vi "FSK - TESTBENCH2.vi"() -> ()   [LabVIEW 2013]
uses:
  Object/FSK_OBJ - PROP.ctl
  <vilib>/sound2/lvsound2.llb/Sampling Mode.ctl
  <vilib>/sound2/lvsound2.llb/Sound Data Format.ctl
  <vilib>/sound2/lvsound2.llb/Sound Output Write (DBL Single).vi
  <vilib>/Analysis/NI_AALPro.lvlib
  <vilib>/Analysis/NI_AALBase.lvlib
panel:
  in  "String":string="KD0QJP >> test"
  out "Array":u8[](array[numeric])
  out "x+y":dbl[](array[numeric])
  in  "PROPERTIES":T1={"rate (bit/s)"=128.0, "bp (Bit Period)"=1e-06, "f1%"=80.0, "f2%"=20.0, "f1 (1 Freq)"=0.0, "f2 (0 Freq)"=0.0, "t (Time arry)"=[], "y1 (f1 cos arry)"=[], "y2 (f2 cos arry)"=[], "data length (B)"=0, "data size"=0, "sample size"=0.0} {"f2%" format="%#_6f"; "f1%" format="%#_6f"; "sample size" format="%#_13g"; "y2 (f2 cos arry)" format="%#_6f"; "y1 (f1 cos arry)" format="%#_6f"; "t (Time arry)" format="%#_6f"; "f2 (0 Freq)" format="%#_6f"; "f1 (1 Freq)" format="%#_6f"; "bp (Bit Period)" format="%#_13f"; "rate (bit/s)" format="%#_13g"}
  in  "rate (bit/s)":dbl=128.0 format="%#_13g"
  out "x-y":u32=9198
  out "demodulated 2":dbl[](graph)
  in  "noise":dbl format="%#_13g"
  out "samples":dbl=344.53125 format="%#_13g"
  in  "data length (B)":i32=100
  out "demodulated":i16[][](graph)
  out "y1":dbl[](array[numeric])=[0.9893761484577952, 0.9577303262743624, 0.9057349344833171, 0.8344947557311932, 0.7455234801837959, 0.6407115430869976, 0.5222859573599328, 0.3927629946857276, 0.2548947205178964, 0.11161051901071738, -0.03404514966549826, -0.17897743711015687, -0.32010686511229053, -0.454434757489237, -0.5791069550678165, -0.6914744600109982, -0.789149720937414, -0.870057362904207, -0.9324782843576068, -0.9750861840923166, -0.9969757421057228, -0.9976818555685076, -0.9771895211914697, -0.9359341540109593, -0.8747923358194655, -0.7950631898159626, -0.6984407772219063, -0.5869781023713945, -0.46304349108464504, -0.32927026918416136, -0.18850081036952815, -0.04372614230499255, 0.10197760584826618, 0.24551456411120198, 0.38383490181300384, 0.5139996294876503, 0.6332430456494466, 0.7390315015970159, 0.8291172356286265, 0.901586132815433, 0.9548983955471564, 0.9879212606945145, 0.9999530682238599, 0.99073816986124, 0.9604723610310173, 0.9097987206528254, 0.8397939471916264, 0.7519454812884151, 0.6481199010631241, 0.5305232616169475, 0.40165422142856066, 0.26425095160066, 0.12123295601337575, -0.024360961427325113, -0.16943726439276915, -0.31091341467296013, -0.44578336903321847, -0.5711814507282928, -0.68444323855097, -0.7831621796627842, -0.8652407233141844, -0.928934888980065, -0.9728913219401479, -0.9961760489582477, -0.9982943230682821, -0.9792011358109098, -0.9393021735599112, -0.8794451976185704, -0.8009020312392202, -0.7053415363003983, -0.5947941538251642, -0.4716087617731102, -0.33840276677889497, -0.19800649027321907, -0.0534030306534317, 0.09233512070548741, 0.23611136283539147, 0.37487078083291553, 0.505665055784281, 0.6257151097701805, 0.7324701548882544, 0.8236618916370709, 0.8973527050704397, 0.9519768346644794, 0.9863736431323324, 0.9998122773006225, 0.992007197060682, 0.9631242424399986, 0.9137771098825537, 0.8450143126089946, 0.7582969021190435, 0.6554674242030396, 0.538710769076067, 0.4105077474793923, 0.27358237915042416, 0.13084401366014314, -0.014674486582761001, -0.15988118769183848, -0.30169078079605705, -0.4370901377666174, -0.5632023332687892, -0.6773477728172205, -0.7771011280039442, -0.8603428691562804, -0.9253043004739954, -0.9706051407525118, -0.9952828511881177, -0.9988130871166739, -0.9811208391333528, -0.9425820268702003, -0.884015511567408, -0.8066656971528188, -0.7121760895167505, -0.6025543757868123, -0.48012976558794696, -0.34750350068787894, -0.2074935845844053, -0.06307490640375905, 0.0826839686602312, 0.22668599930828476, 0.36587147314964674, 0.49728301856246626, 0.6181284420479548, 0.7258400559287772, 0.8181292358144563, 0.8930350486128749, 0.9489659178543944, 0.9847334410361209, 0.9995776404454229, 0.993183110940726, 0.9656857215863112, 0.917669728746776, 0.8501553619812785, 0.764577146508786, 0.6627534228421479, 0.5468477112287864, 0.41932274181484397, 0.2828881272862825, 0.14044278982303418, -0.004986634338720148, -0.1503101039746513, -0.2924398291507459, -0.4283558796669867, -0.5551703516376055, -0.6701887288153613, -0.7709671348727278, -0.8553642601604833, -0.9215868596193315, -0.9682278551184964, -0.9942962326340482, -0.9992380990206453, -0.9829484509686218, -0.9457734060831376, -0.8885028486800673, -0.8123536465585929, -0.7189437953555021, -0.6102580398543219, -0.48860570271744064, -0.3565716166838698, -0.2169612028106756, -0.07274086171932041, 0.07302505560394744, 0.21723935822802365, 0.35683782347021975, 0.4888543045900402, 0.6104837545943896, 0.719141827043265, 0.812519787475543, 0.8886335687133354, 0.9458659277322674, 0.9830008083610837, 0.99924917968211, 0.9942658011259113, 0.9681565580404066, 0.921476211870435, 0.8552166127512957, 0.7707856249715608, 0.6699772130907016, 0.5549333243127685, 0.42809837702819653, 0.29216732253760874, 0.15002838352677486, 0.004701685968533666, -0.14072491161716658, -0.28316142806424205, -0.4195814145628546, -0.547086259745096, -0.6629667785187164, -0.7647607760275437, -0.8503053636367329, -0.91778291534829, -0.9657596881785818, -0.9932162859035644, -0.9995693188870678, -0.9846837997705735, -0.9488760116445256, -0.8929067877591376, -0.8179653455653881, -0.7256440185757311, -0.617904422934397, -0.49703577758001233, -0.365606263601276, -0.22640845628773937, -0.0823999893192048, 0.06335928815654623, 0.20777232628990394, 0.34777067972510023, 0.48037970501603106, 0.6027817649670083, 0.71237609695127, 0.8068340731430783, 0.88414867851036, 0.9426771552741793, 0.9811759077382782, 0.9988269258411779, 0.9952551659910911, 0.9705365198808007, 0.9251962019635079, 0.8601975898520701, 0.7769217547575329, 0.6771381168980871, 0.5629668493836544, 0.4368338294071522, 0.3014190939261879, 0.15959989503350175, 0.014389564958840763, -0.13112651031957948, -0.27385644844022766, -0.41076756605667397, -0.5389508163928424, -0.6556825998051955, -0.7584826340192738, -0.8451666544310259, -0.9138928247125881, -0.9632008716036847, -0.9920431123643015, -0.999806715626468, -0.9863267226532054, -0.9518895523327884, -0.8972269154352526, -0.8235002674392077, -0.7322761302706873, -0.6254928073103707, -0.5054191988988894, -0.37460659341604435, -0.23583445826283292, -0.09205138256338727, 0.05368757358128155, 0.1982857921031729, 0.33867089298859904, 0.4718600152964715, 0.5950231961019138, 0.7055435007082523, 0.8010726264984068, 0.879580798971675, 0.939399899789645, 0.9792589104593589, 0.9983109185568722, 0.9961511126709647, 0.9728253837158201, 0.9288293498545073, 0.8650978257513989, 0.7829849599077564, 0.6842354621164354, 0.5709475323862405, 0.4455282790111326, 0.3106425730478823, 0.1691564259271335, 0.02407609329346504, -0.12151580102193553, -0.26452576367715097, -0.40191516144758455, -0.5307647852024573, -0.6483368763936876, -0.7521332981366267, -0.839948614880866, -0.9099169528499557, -0.9605516455734184, -0.990776822134496, -0.9999502669559449, -0.9878770654059384, -0.9548137452862886, -0.9014628262058824, -0.8289578926526208, -0.738839507926803, -0.633022480709521, -0.5137551797763668, -0.3835717613252466, -0.2452383239779305, -0.1016941355378064, 0.04401081969965071, 0.18878064610762815, 0.3295393173990277, 0.4632960351196873, 0.5872087762459463, 0.6986446796459717, 0.7952359883313769, 0.87493035885468, 0.9360344688935001, 0.9772499964605014, 0.9977012062634695, 0.9969535570687938, 0.9750229347045744, 0.9323753145232648, 0.8699168604957301, 0.7889746713082603, 0.6912685825637127, 0.5788746242252764, 0.45418090974819686, 0.31983689415418065, 0.17869707919773656, 0.033760361760447735, -0.11189368581954229, -0.2551702495862256, -0.393025031653726, -0.5225289345439073, -0.6409302977798866, -0.7457133643508318, -0.8346517347699798, -0.9058556729498477, -0.9578122587535489, -0.989417534072646, -0.9999999594012605, -0.9893346825080953, -0.9576483160298892, -0.905614122473395, -0.8343377089335418, -0.7453335354821389, -0.6404927363699581, -0.5220429377676673, -0.39250092582637613, -0.25461917075277707, -0.11132734313941778, 0.034329934806144054, 0.1792577804900378, 0.32037681007850216, 0.4546885683312952, 0.5793392388883094, 0.691680281312277, 0.7893247064895802, 0.8701977946662005, 0.9325811784770495, 0.9751493543055092, 0.9969978461907315, 0.9976624238642972]
  out "y2":dbl[](array[numeric])=[0.999334903985156, 0.997340500646042, 0.9940194429220834, 0.9893761484577952, 0.983416793726465, 0.9761493058142584, 0.9675833518756722, 0.9577303262743624, 0.9466033354264518, 0.9342171803664809, 0.920588337059189, 0.9057349344833171, 0.8896767305165856, 0.8724350856539221, 0.8540329345939015, 0.8344947557311932, 0.8138465385955947, 0.7921157492809673, 0.769331293910056, 0.7455234801837959, 0.7207239770662501, 0.6949657726588057, 0.6682831303196646, 0.6407115430869973, 0.6122876864663866, 0.5830493696453622, 0.5530354851999211, 0.5222859573599322, 0.49084168890224517, 0.458744506742142, 0.4260371062955071, 0.3927629946857266, 0.3589664328708588, 0.3246923767680605, 0.2899864174535852, 0.25489472051789513, 0.21946396465656262, 0.1837412795786402, 0.1477741833150976, 0.11161051901071582, 0.07529839128351644, 0.0388861022363834, 0.002422087205989877, -0.034045149665500256, -0.07046709995025559, -0.10679531546030208, -0.14298147269291528, -0.1789774371101593, -0.2147353271670654, -0.2502075780032812, -0.2853470047134697, -0.320106865112293, -0.3544409219104956, -0.3883035042193773, -0.4216495683018469, -0.4544347574892398, -0.4866154611842069, -0.5181488728711843, -0.5489930470572765, -0.5791069550678191, -0.6084505396223935, -0.6369847681187029, -0.6646716845534281, -0.6914744600110011, -0.7173574416531345, -0.7422862001439438, -0.7662275754475737, -0.7891497209374164, -0.8110221457582377, -0.831815755384871, -0.8515028903235224, -0.8700573629042091, -0.8874544921153893, -0.9036711364344469, -0.9186857246103601, -0.9324782843576086, -0.9450304689231472, -0.9563255814911122, -0.966348597392791, -0.9750861840923176, -0.9825267189215059, -0.9886603045402291, -0.9934787821017842, -0.9969757421057232, -0.9991465329237209, -0.9999882669871332, -0.9994998246280177, -0.9976818555685074, -0.9945367780565556, -0.9900687756492015, -0.9842837916476358, -0.9771895211914694, -0.9687954010227195, -0.9591125969331309, -0.9481539889115284, -0.9359341540109589, -0.9224693469584113, -0.9077774785329082, -0.8918780917407305, -0.8747923358194658, -0.856542938105462, -0.8371541738021047, -0.8166518336891359, -0.7950631898159637, -0.7724169592246001, -0.7487432657504801, -0.7240735999519763, -0.6984407772219086, -0.6718788941367715, -0.6444232831017385, -0.6161104653517774, -0.5869781023713981, -0.5570649457976438, -0.5264107858729701, -0.4950563985165871, -0.4630434910846506, -0.4304146468914752, -0.39721326856554295, -0.3634835203156785, -0.3292702691841681, -0.2946190253649748, -0.25957588166644746, -0.22418745219902733, -0.18850081036953686, -0.15256342626450223, -0.11642310350582868, -0.08012791566280102, -0.043726142305002304, -0.00726620478122136, 0.029203398190246532, 0.06563415503420107, 0.1019776058482547, 0.13818540686380232, 0.17420939475251962, 0.21000165069284124, 0.24551456411118905, 0.2807008960131847, 0.3155138418205765, 0.3499070936303232, 0.38383490181299157, 0.41725213586855137, 0.4501143444586093, 0.4823778145352195, 0.5139996294876373, 0.5449377262296482, 0.5751509511515512, 0.6045991148623658, 0.6332430456494335, 0.6610446415843235, 0.6879669212057095, 0.7139740727118193, 0.7390315015970039, 0.7631058766690754, 0.7861651743861942, 0.8081787214543256, 0.8291172356286155, 0.8489528646643949, 0.8676592233660174, 0.8852114286842332, 0.9015861328154241, 0.9167615542586671, 0.9307175067893105, 0.943435426310532, 0.9548983955471497, 0.9650911665488493, 0.9740001809728829, 0.9816135881192718, 0.9879212606945109, 0.9929148082828151, 0.9965875885069823, 0.9989347158640314, 0.9999530682238595, 0.9996412909822744, 0.9979997988628776, 0.9950307753654032, 0.9907381698612435, 0.9851276923400267, 0.9782068058142344, 0.9699847163919613, 0.9604723610310247, 0.9496823929907088, 0.9376291650005016, 0.9243287101682082, 0.9097987206528368, 0.8940585241306331, 0.8771290580855559, 0.8590328419584059, 0.8397939471916422, 0.8194379652097441, 0.7979919733777007, 0.7754844989829147, 0.7519454812884356, 0.7274062317079862, 0.7018993921557741, 0.675458891626473, 0.6481199010631484, 0.6199187865731481, 0.5908930610541938, 0.5610813342950279, 0.5305232616169754, 0.49925949112475654, 0.4673316096366968, 0.43478208736627705, 0.40165422142859236, 0.367992078246872, 0.3338404349356802, 0.2992447197387486, 0.2642509516006951, 0.22890567895298405, 0.1932559177955794, 0.15734908915663393, 0.12123295601341277, 0.08495555975836794, 0.04856515629485395, 0.012110151847516893, -0.024360961427286932, -0.06079966994536465, -0.09715750322707249, -0.13338609837236418, -0.1694372643927289, -0.20526304631446715, -0.24081578896800843, -0.2760482003784414, -0.3109134146729196, -0.3453650544212785, -0.37935729232691345, -0.41284491218589114, -0.44578336903318033, -0.4781288483960157, -0.5098383245755508, -0.5408696178793061, -0.5711814507282579, -0.6007335025639439, -0.6294864634825542, -0.6574020865246436, -0.6844432385509376, -0.7105739496365373, -0.7357594609178254, -0.7599662708284343, -0.7831621796627555, -0.8053163324077363, -0.8263992597859696, -0.8463829174554968, -0.8652407233141605, -0.8829475928589102, -0.8994799725530068, -0.9148158711567487, -0.9289348889800466, -0.9418182450179241, -0.9534488019328641, -0.9638110888507574, -0.9728913219401361, -0.9806774227473178, -0.9871590342630662, -0.9923275346994032, -0.9961760489582432, -0.9986994577765927, -0.9998944045361543, -0.9997592997282723, -0.9982943230682852, -0.9955014232564702, -0.9913843153858962, -0.9859484760006382, -0.979201135810921, -0.9711512700748869, -0.9618095866597781, -0.9511885117984167, -0.9393021735599301, -0.9261663830567055, -0.911798613412574, -0.8962179765202013, -0.8794451976185975, -0.8615025877245741, -0.8424140139548039, -0.8222048677779745, -0.8009020312392553, -0.7785338412020207, -0.7551300516543767, -0.7307217941306443, -0.7053415363004412, -0.6790230387804421, -0.6518013102262827, -0.6237125607643202, -0.5947941538252127, -0.5650845564433834, -0.5346232880884718, -0.5034508680968593, -0.471608761773165, -0.4391393252334305, -0.40608574906334644, -0.37249200086648837, -0.33840276677895514, -0.3038633920282282, -0.2689198206153131, -0.23361853420038867, -0.1980064902732835, -0.1621310596909903, -0.12603996366533124, -0.0897812102845842, -0.053403030653499106, -0.016953814736677533, 0.019517953009379575, 0.05596375812990778, 0.09233512070541842, 0.12858365983930822, 0.16466115801373166, 0.20051962522816602, 0.23611136283532413, 0.27138902698952166, 0.306305691623073, 0.3408149108669792, 0.3748707808328513, 0.40842800067389506, 0.4414419328437426, 0.47386866247295134, 0.5056650557842197, 0.5367888174685921, 0.5671985469463406, 0.5968537934376921, 0.6257151097701237, 0.6537441048506837, 0.6809034947335145, 0.7071571522146655, 0.7324701548882036, 0.7568088315997251, 0.7801408072354551, 0.8024350457873651, 0.8236618916370276, 0.8437931090032768, 0.8628019195012241, 0.8806630377626514, 0.8973527050704053, 0.9128487209620563, 0.9271304727607728, 0.9401789629941419, 0.9519768346644555, 0.9625083943368513, 0.9717596330145924, 0.9797182447737252, 0.9863736431323198, 0.9917169751325254, 0.9957411331167036, 0.9984407641819776, 0.999812277300621, 0.9998538480968151]
  out "size(s)":i32=276000
  out "m":dbl[](graph)
  out "t2":dbl[](array[numeric])=[2.9024943310657594e-09, 5.804988662131519e-09, 8.707482993197278e-09, 1.1609977324263038e-08, 1.4512471655328797e-08, 1.7414965986394556e-08, 2.0317460317460316e-08, 2.3219954648526075e-08, 2.6122448979591834e-08, 2.9024943310657594e-08, 3.192743764172335e-08, 3.482993197278911e-08, 3.773242630385487e-08, 4.063492063492063e-08, 4.353741496598639e-08, 4.643990929705215e-08, 4.934240362811791e-08, 5.224489795918367e-08, 5.514739229024943e-08, 5.804988662131519e-08, 6.095238095238095e-08, 6.385487528344672e-08, 6.675736961451249e-08, 6.965986394557825e-08, 7.256235827664402e-08, 7.546485260770978e-08, 7.836734693877555e-08, 8.126984126984132e-08, 8.417233560090708e-08, 8.707482993197285e-08, 8.997732426303861e-08, 9.287981859410438e-08, 9.578231292517015e-08, 9.868480725623591e-08, 1.0158730158730168e-07, 1.0448979591836744e-07, 1.0739229024943321e-07, 1.1029478458049898e-07, 1.1319727891156474e-07, 1.1609977324263051e-07, 1.1900226757369627e-07, 1.2190476190476204e-07, 1.248072562358278e-07, 1.2770975056689357e-07, 1.3061224489795934e-07, 1.335147392290251e-07, 1.3641723356009087e-07, 1.3931972789115664e-07, 1.422222222222224e-07, 1.4512471655328817e-07, 1.4802721088435393e-07, 1.509297052154197e-07, 1.5383219954648547e-07, 1.5673469387755123e-07, 1.59637188208617e-07, 1.6253968253968276e-07, 1.6544217687074853e-07, 1.683446712018143e-07, 1.7124716553288006e-07, 1.7414965986394583e-07, 1.770521541950116e-07, 1.7995464852607736e-07, 1.8285714285714313e-07, 1.857596371882089e-07, 1.8866213151927466e-07, 1.9156462585034042e-07, 1.944671201814062e-07, 1.9736961451247196e-07, 2.0027210884353772e-07, 2.031746031746035e-07, 2.0607709750566925e-07, 2.0897959183673502e-07, 2.1188208616780079e-07, 2.1478458049886655e-07, 2.1768707482993232e-07, 2.2058956916099808e-07, 2.2349206349206385e-07, 2.2639455782312962e-07, 2.2929705215419538e-07, 2.3219954648526115e-07, 2.3510204081632691e-07, 2.3800453514739268e-07, 2.4090702947845845e-07, 2.438095238095242e-07, 2.467120181405899e-07, 2.4961451247165566e-07, 2.525170068027214e-07, 2.5541950113378714e-07, 2.583219954648529e-07, 2.612244897959186e-07, 2.6412698412698436e-07, 2.670294784580501e-07, 2.6993197278911584e-07, 2.728344671201816e-07, 2.757369614512473e-07, 2.7863945578231306e-07, 2.815419501133788e-07, 2.8444444444444454e-07, 2.873469387755103e-07, 2.90249433106576e-07, 2.9315192743764176e-07, 2.960544217687075e-07, 2.9895691609977324e-07, 3.01859410430839e-07, 3.047619047619047e-07, 3.0766439909297045e-07, 3.105668934240362e-07, 3.1346938775510193e-07, 3.1637188208616767e-07, 3.192743764172334e-07, 3.2217687074829915e-07, 3.250793650793649e-07, 3.2798185941043063e-07, 3.3088435374149637e-07, 3.337868480725621e-07, 3.3668934240362785e-07, 3.395918367346936e-07, 3.4249433106575933e-07, 3.4539682539682507e-07, 3.482993197278908e-07, 3.5120181405895655e-07, 3.541043083900223e-07, 3.5700680272108803e-07, 3.5990929705215377e-07, 3.628117913832195e-07, 3.6571428571428525e-07, 3.68616780045351e-07, 3.715192743764167e-07, 3.7442176870748246e-07, 3.773242630385482e-07, 3.8022675736961394e-07, 3.831292517006797e-07, 3.860317460317454e-07, 3.8893424036281116e-07, 3.918367346938769e-07, 3.9473922902494264e-07, 3.976417233560084e-07, 4.005442176870741e-07, 4.0344671201813986e-07, 4.063492063492056e-07, 4.0925170068027134e-07, 4.121541950113371e-07, 4.150566893424028e-07, 4.1795918367346856e-07, 4.208616780045343e-07, 4.2376417233560004e-07, 4.266666666666658e-07, 4.295691609977315e-07, 4.3247165532879725e-07, 4.35374149659863e-07, 4.3827664399092873e-07, 4.4117913832199447e-07, 4.440816326530602e-07, 4.4698412698412595e-07, 4.498866213151917e-07, 4.5278911564625743e-07, 4.5569160997732317e-07, 4.585941043083889e-07, 4.6149659863945465e-07, 4.643990929705204e-07, 4.6730158730158613e-07, 4.7020408163265187e-07, 4.731065759637176e-07, 4.7600907029478335e-07, 4.789115646258491e-07, 4.818140589569149e-07, 4.847165532879806e-07, 4.876190476190464e-07, 4.905215419501121e-07, 4.934240362811778e-07, 4.963265306122436e-07, 4.992290249433093e-07, 5.021315192743751e-07, 5.050340136054408e-07, 5.079365079365065e-07, 5.108390022675723e-07, 5.13741496598638e-07, 5.166439909297038e-07, 5.195464852607695e-07, 5.224489795918352e-07, 5.25351473922901e-07, 5.282539682539667e-07, 5.311564625850325e-07, 5.340589569160982e-07, 5.369614512471639e-07, 5.398639455782297e-07, 5.427664399092954e-07, 5.456689342403611e-07, 5.485714285714269e-07, 5.514739229024926e-07, 5.543764172335584e-07, 5.572789115646241e-07, 5.601814058956898e-07, 5.630839002267556e-07, 5.659863945578213e-07, 5.688888888888871e-07, 5.717913832199528e-07, 5.746938775510185e-07, 5.775963718820843e-07, 5.8049886621315e-07, 5.834013605442158e-07, 5.863038548752815e-07, 5.892063492063472e-07, 5.92108843537413e-07, 5.950113378684787e-07, 5.979138321995445e-07, 6.008163265306102e-07, 6.037188208616759e-07, 6.066213151927417e-07, 6.095238095238074e-07, 6.124263038548732e-07, 6.153287981859389e-07, 6.182312925170046e-07, 6.211337868480704e-07, 6.240362811791361e-07, 6.269387755102019e-07, 6.298412698412676e-07, 6.327437641723333e-07, 6.356462585033991e-07, 6.385487528344648e-07, 6.414512471655306e-07, 6.443537414965963e-07, 6.47256235827662e-07, 6.501587301587278e-07, 6.530612244897935e-07, 6.559637188208593e-07, 6.58866213151925e-07, 6.617687074829907e-07, 6.646712018140565e-07, 6.675736961451222e-07, 6.70476190476188e-07, 6.733786848072537e-07, 6.762811791383194e-07, 6.791836734693852e-07, 6.820861678004509e-07, 6.849886621315166e-07, 6.878911564625824e-07, 6.907936507936481e-07, 6.936961451247139e-07, 6.965986394557796e-07, 6.995011337868453e-07, 7.024036281179111e-07, 7.053061224489768e-07, 7.082086167800426e-07, 7.111111111111083e-07, 7.14013605442174e-07, 7.169160997732398e-07, 7.198185941043055e-07, 7.227210884353713e-07, 7.25623582766437e-07, 7.285260770975027e-07, 7.314285714285685e-07, 7.343310657596342e-07, 7.372335600907e-07, 7.401360544217657e-07, 7.430385487528314e-07, 7.459410430838972e-07, 7.488435374149629e-07, 7.517460317460287e-07, 7.546485260770944e-07, 7.575510204081601e-07, 7.604535147392259e-07, 7.633560090702916e-07, 7.662585034013574e-07, 7.691609977324231e-07, 7.720634920634888e-07, 7.749659863945546e-07, 7.778684807256203e-07, 7.80770975056686e-07, 7.836734693877518e-07, 7.865759637188175e-07, 7.894784580498833e-07, 7.92380952380949e-07, 7.952834467120147e-07, 7.981859410430805e-07, 8.010884353741462e-07, 8.03990929705212e-07, 8.068934240362777e-07, 8.097959183673434e-07, 8.126984126984092e-07, 8.156009070294749e-07, 8.185034013605407e-07, 8.214058956916064e-07, 8.243083900226721e-07, 8.272108843537379e-07, 8.301133786848036e-07, 8.330158730158694e-07, 8.359183673469351e-07, 8.388208616780008e-07, 8.417233560090666e-07, 8.446258503401323e-07, 8.475283446711981e-07, 8.504308390022638e-07, 8.533333333333295e-07, 8.562358276643953e-07, 8.59138321995461e-07, 8.620408163265268e-07, 8.649433106575925e-07, 8.678458049886582e-07, 8.70748299319724e-07, 8.736507936507897e-07, 8.765532879818555e-07, 8.794557823129212e-07, 8.823582766439869e-07, 8.852607709750527e-07, 8.881632653061184e-07, 8.910657596371842e-07, 8.939682539682499e-07, 8.968707482993156e-07, 8.997732426303814e-07, 9.026757369614471e-07, 9.055782312925129e-07, 9.084807256235786e-07, 9.113832199546443e-07, 9.142857142857101e-07, 9.171882086167758e-07, 9.200907029478415e-07, 9.229931972789073e-07, 9.25895691609973e-07, 9.287981859410388e-07, 9.317006802721045e-07, 9.346031746031702e-07, 9.37505668934236e-07, 9.404081632653017e-07, 9.433106575963675e-07, 9.462131519274332e-07, 9.491156462584989e-07, 9.520181405895647e-07, 9.549206349206304e-07, 9.578231292516962e-07, 9.60725623582762e-07, 9.636281179138276e-07, 9.665306122448934e-07, 9.694331065759591e-07, 9.723356009070249e-07, 9.752380952380906e-07, 9.781405895691563e-07, 9.81043083900222e-07, 9.839455782312878e-07, 9.868480725623536e-07, 9.897505668934193e-07, 9.92653061224485e-07, 9.955555555555508e-07, 9.984580498866165e-07, 1.0013605442176823e-06] format="%#_6f"
  out "ss":i32=345
  out "f2 (0 Freq)":dbl=2000000.0 format="%#_6f"
  out "f1 (1 Freq)":dbl=8000000.0 format="%#_6f"
  out "br (Bit Rate)":dbl=1000000.0 format="%#_6f"
  in  "bp (Bit Period)":dbl=1e-06 format="%#_13f"
  # "ss=700, data=100, time=25000 rate=32 bit/s\nss=700, data=50,   time=13000 rate=31 bit/s \nss=440, data=100, time=8000   rate=100 bit/s\nss=100, data=100, time=2000   rate=400 bit/s\nss=10000, data=100, time=183000, rate=4.3 bit/s\nss=1000, data=100, time=18500, rate=43 bit/s"
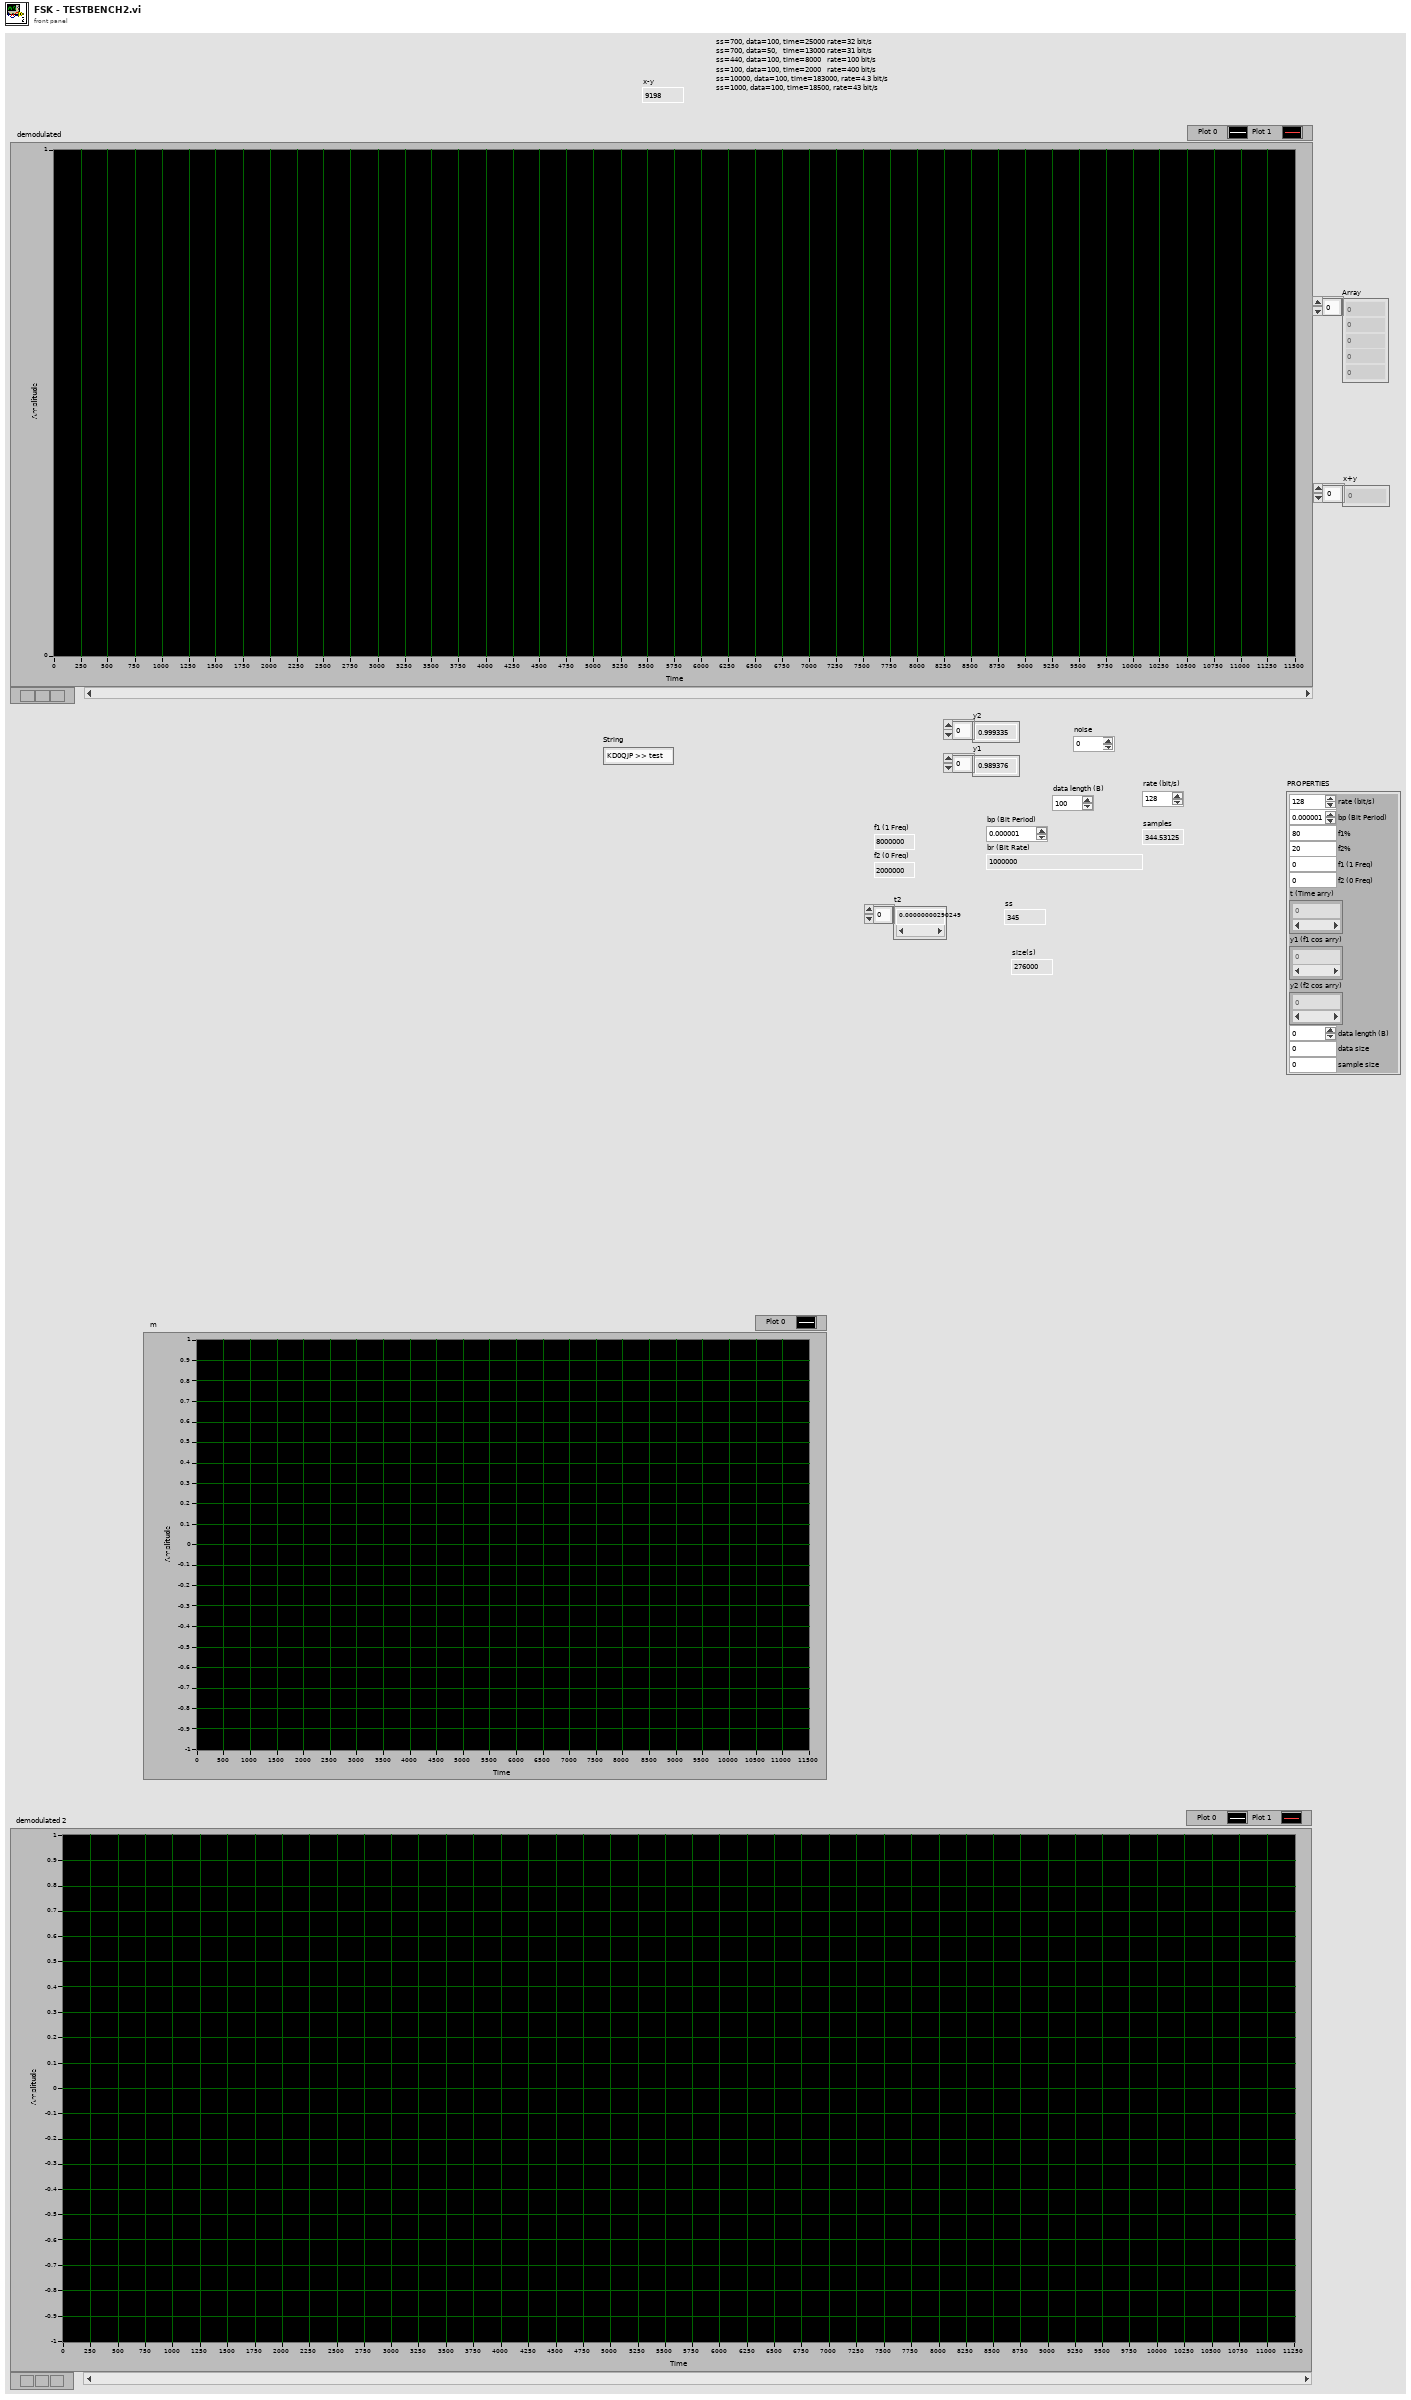
[diagram p1: front panel]
types:
  T1 = typedef "FSK_OBJ - PROP.ctl" = cluster{"rate (bit/s)":dbl, "bp (Bit Period)":dbl, "f1%":dbl, "f2%":dbl, "f1 (1 Freq)":dbl, "f2 (0 Freq)":dbl, "t (Time arry)":dbl[], "y1 (f1 cos arry)":dbl[], "y2 (f2 cos arry)":dbl[], "data length (B)":i32, "data size":i32, "sample size":dbl}
  T2 = typedef "Sound Data Format.ctl" = cluster{"sample rate (S/s)":dbl, "number of channels":i32, "bits per sample":i32}
  T3 = typedef "Sampling Mode.ctl" = i32
  T4 = typedef "Sound Output Task ID.ctl" = u32
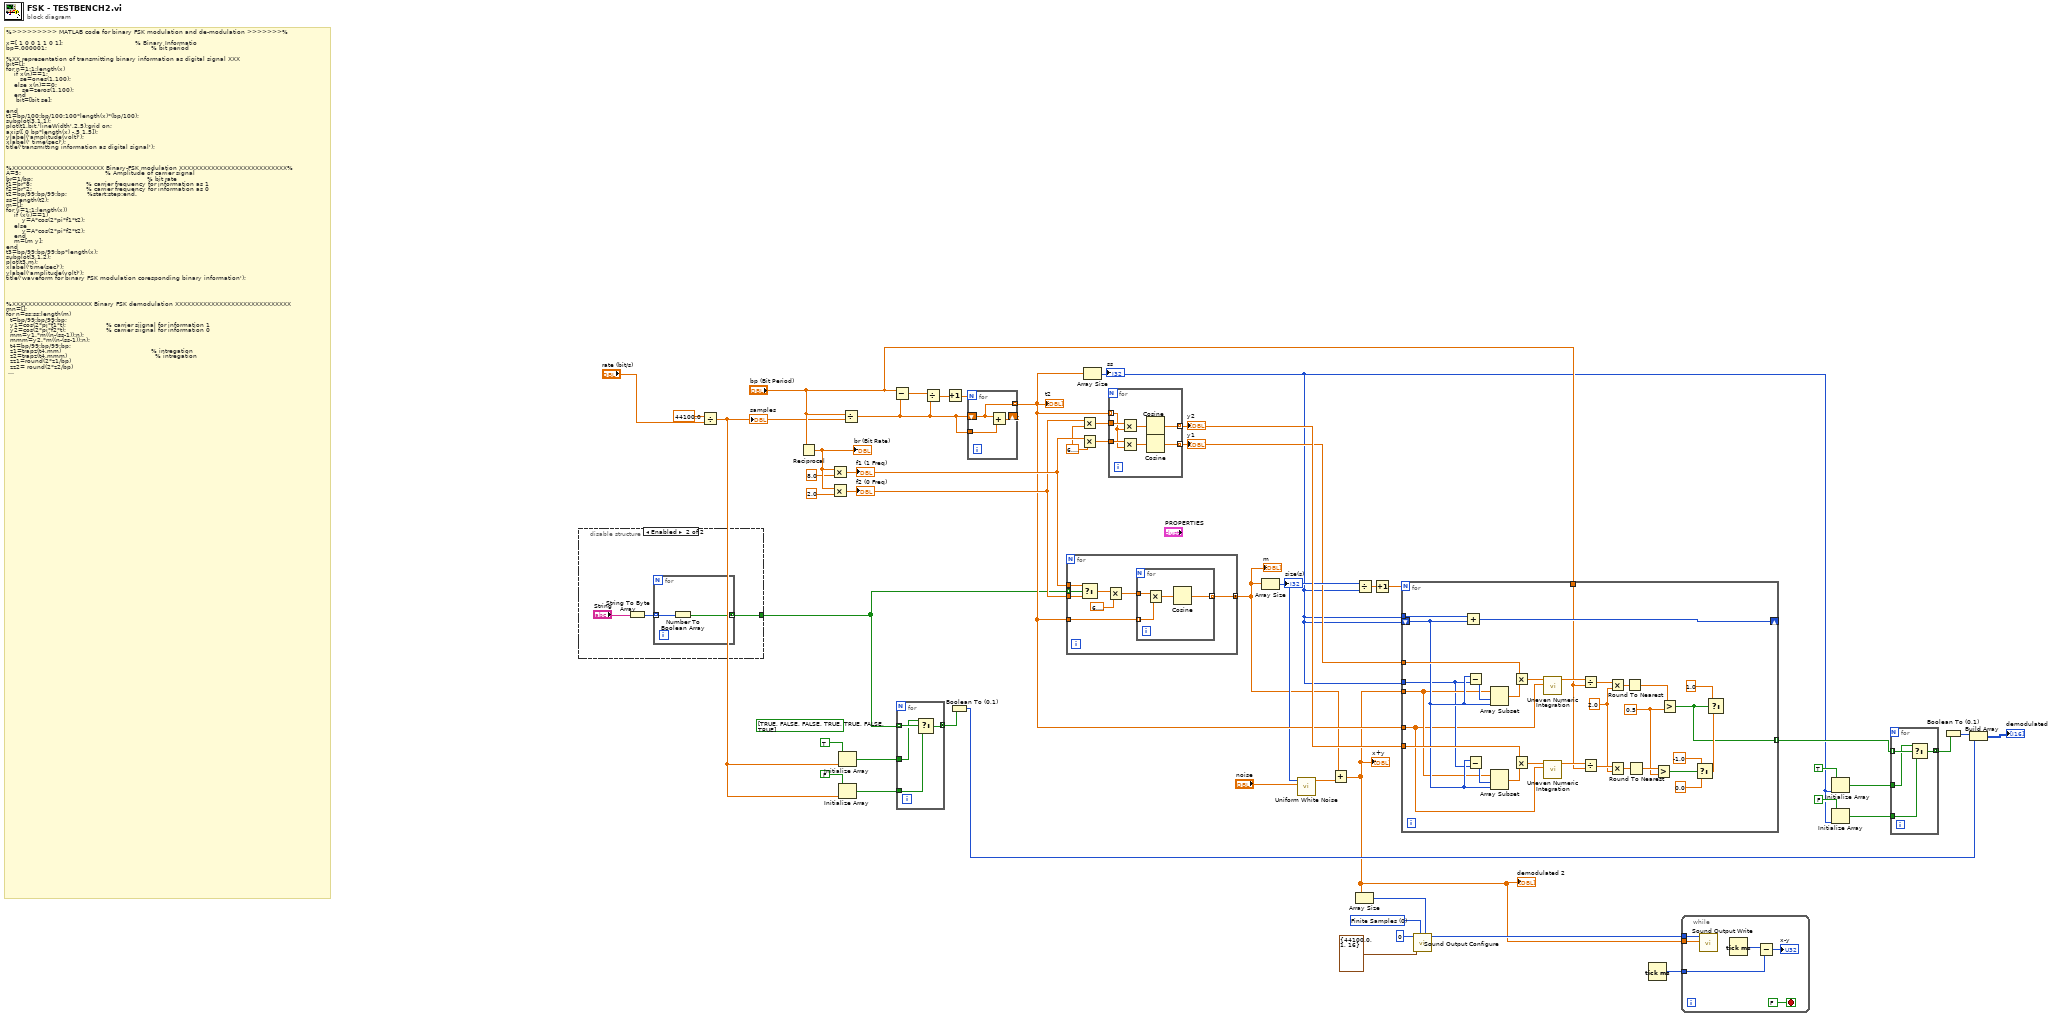
[diagram p0: block diagram]
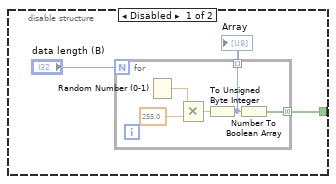
[diagram p2: hidden frame]
diagram:
  w23 = T3 0 items=["Finite Samples", "Continuous Samples"] ("sample mode")
  w34 = 6.283185307179586
  (unwired) bool[] [TRUE, FALSE, FALSE, TRUE, TRUE, FALSE, TRUE]
  # "%>>>>>>>>> MATLAB code for binary FSK modulation and de-modulation >>>>>>>%\n\nx=[ 1 0 0 1 1 0 1];                                    % Binary Informatio\nbp=.000001;                                                    % bit period\n\n%XX representation of transmitting binary information as digital signal XXX\nbit=[]; \nfor n=1:1:length(x)\n    if x(n)==1;\n       se=ones(1,100);\n    else x(n)==0;\n        se=zeros(1,100);\n    end\n     bit=[bit se];\n\nend\nt1=bp/100:bp/100:100*length(x)*(bp/100);\nsubplot(3,1,1);\nplot(t1,bit,'lineWidth',2.5);grid on;\naxis([ 0 bp*length(x) -.5 1.5]);\nylabel('amplitude(volt)');\nxlabel(' time(sec)');\ntitle('transmitting information as digital signal');\n\n\n\n%XXXXXXXXXXXXXXXXXXXXXXX Binary-FSK modulation XXXXXXXXXXXXXXXXXXXXXXXXXXX%\nA=5;                                          % Amplitude of carrier signal\nbr=1/bp;                                                         % bit rate\nf1=br*8;                           % carrier frequency for information as 1\nf2=br*2;                           % carrier frequency for information as 0\nt2=bp/99:bp/99:bp;          %start:step:end.       \nss=length(t2);\nm=[];\nfor (i=1:1:length(x))\n    if (x(i)==1)\n        y=A*cos(2*pi*f1*t2);\n    else\n        y=A*cos(2*pi*f2*t2);\n    end\n    m=[m y];\nend\nt3=bp/99:bp/99:bp*length(x);\nsubplot(3,1,2);\nplot(t3,m);\nxlabel('time(sec)');\nylabel('amplitude(volt)');\ntitle('waveform for binary FSK modulation coresponding binary information');\n\n\n\n\n%XXXXXXXXXXXXXXXXXXXX Binary FSK demodulation XXXXXXXXXXXXXXXXXXXXXXXXXXXXX\nmn=[];\nfor n=ss:ss:length(m)\n  t=bp/99:bp/99:bp;\n  y1=cos(2*pi*f1*t);                    % carrier siignal for information 1\n  y2=cos(2*pi*f2*t);                    % carrier siignal for information 0\n  mm=y1.*m((n-(ss-1)):n);\n  mmm=y2.*m((n-(ss-1)):n);\n  t4=bp/99:bp/99:bp;\n  z1=trapz(t4,mm)                                             % intregation \n  z2=trapz(t4,mmm)                                            % intregation \n  zz1=round(2*z1/bp)\n  zz2= round(2*z2/bp)\n  if(zz1>A/2)      % logic lavel= (0+A)/2 or (A+0)/2 or 2.5 ( in this case)\n    a=1;\n  else(zz2>A/2)\n    a=0;\n  end\n  mn=[mn a];\nend\ndisp(' Binary information at Reciver :');\ndisp(mn);\n\n\n%XXXXX Representation of binary information as digital signal which achived \n%after demodulation XXXXXXXXXXXXXXXXXXXXXXXXXXXXXXXXXXXXXXXXXXXXXXXXXXXXXXX\nbit=[];\nfor n=1:length(mn);\n    if mn(n)==1;\n       se=ones(1,100);\n    else mn(n)==0;\n        se=zeros(1,100);\n    end\n     bit=[bit se];\n\nend\nt4=bp/100:bp/100:100*length(mn)*(bp/100);\nsubplot(3,1,3)\nplot(t4,bit,'LineWidth',2.5);grid on;\naxis([ 0 bp*length(mn) -.5 1.5]);\nylabel('amplitude(volt)');\nxlabel(' time(sec)');\ntitle('recived information as digital signal after binary FSK demodulation');\n\n\n\n%>>>>>>>>>>>>>>>>>>>>>>>>>> end of program >>>>>>>>>>>>>>>>>>>>>>>>>>>>>>%"
  n1 = disable-structure shown="Enabled" {
    disable-tunnel: [w50 w57] -> w13
    frame Disabled {
      n2 = for {
        N: "data length (B)" -> [_]
        tunnel: [w53] -> w50 mode=concatenating
        tunnel: [w52] -> w49 mode=indexing
        n3 = Random Number (0-1)() -> (number: 0 to 1=w56:dbl)
        n4 = Multiply(x=w56, y=255.0) -> (x*y=w54:dbl)
        n5 = To Unsigned Byte Integer(number=w54) -> (unsigned 8bit integer=w52:u8)
        n6 = Number To Boolean Array(number=w52) -> (Boolean array=w53:bool[])
      }
      "Array" <- w49
    }
    frame Enabled {
      n7 = String To Byte Array(string="String") -> (unsigned byte array=w58:u8[])
      n8 = for {
        tunnel: w58 -> [w61] mode=indexing
        tunnel: [w60] -> w57 mode=concatenating
        n9 = Number To Boolean Array(number=w61) -> (Boolean array=w60:bool[])
      }
    }
  }
  n10 = Divide(x=44100.0, y="rate (bit/s)") -> (x/y=w6:dbl)
  "samples" <- w6
  n11 = Reciprocal(x="bp (Bit Period)") -> (1/x=w43:dbl)
  "br (Bit Rate)" <- w43
  n12 = Multiply(x=w43, y=8.0) -> (x*y=w36:dbl)
  "f1 (1 Freq)" <- w36
  n13 = Multiply(x=w43, y=2.0) -> (x*y=w35:dbl)
  "f2 (0 Freq)" <- w35
  n14 = Initialize Array(TRUE, w6) -> (w46:bool[])
  n15 = Initialize Array(FALSE, w6) -> (w45:bool[])
  n16 = Divide(x="bp (Bit Period)", y=w6) -> (x/y=w37:dbl)
  n17 = Subtract(x="bp (Bit Period)", y=w37) -> (x-y=w40:dbl)
  n18 = for {
    tunnel: w13 -> [w65] mode=indexing
    tunnel: w46 -> [w64]
    tunnel: w45 -> [w63]
    tunnel: [w62] -> w44 mode=concatenating
    n19 = Select(t=w64, s=w65, f=w63) -> (s? t:f=w62:bool[])
  }
  n20 = Divide(x=w40, y=w37) -> (x/y=w39:dbl)
  n21 = Increment(x=w39) -> (x+1=w38:dbl)
  n22 = Boolean To (0,1)(Boolean=w44) -> (0, 1=w11:i16[])
  n23 = for {
    N: w38 -> [_]
    shift-right: [w67] -> _
    shift-left: w37 -> [w66]
    tunnel: w37 -> [w68]
    tunnel: [w66] -> w30 mode=indexing
    n24 = Add(x=w66, y=w68) -> (x+y=w67:dbl)
  }
  "t2" <- w30
  n25 = for {
    tunnel: w13 -> [w76] mode=indexing
    tunnel: w30 -> [w70]
    tunnel: w36 -> [w75]
    tunnel: w35 -> [w74]
    tunnel: [w69] -> w25 mode=concatenating
    n26 = Select(t=w75, s=w76, f=w74) -> (s? t:f=w73:dbl)
    n27 = Multiply(x=w73, y=6.283185307179586) -> (x*y=w71:dbl)
    n28 = for {
      tunnel: w71 -> [w80]
      tunnel: w70 -> [w79] mode=indexing
      tunnel: [w77] -> w69 mode=indexing
      n29 = Multiply(x=w80, y=w79) -> (x*y=w78:dbl)
      n30 = Cosine(x=w78) -> (cos(x)=w77:dbl)
    }
  }
  "m" <- w25
  n31 = Multiply(x=w35, y=w34) -> (x*y=w33:dbl)
  n32 = Multiply(x=w36, y=w34) -> (x*y=w32:dbl)
  n33 = Array Size(array=w30) -> (size(s)=w3:i32)
  "ss" <- w3
  n34 = for {
    tunnel: w33 -> [w86]
    tunnel: w32 -> [w87]
    tunnel: w30 -> [w85] mode=indexing
    tunnel: [w82] -> w31 mode=indexing
    tunnel: [w81] -> w7 mode=indexing
    n35 = Multiply(x=w86, y=w85) -> (x*y=w84:dbl)
    n36 = Multiply(x=w87, y=w85) -> (x*y=w83:dbl)
    n37 = Cosine(x=w84) -> (cos(x)=w82:dbl)
    n38 = Cosine(x=w83) -> (cos(x)=w81:dbl)
  }
  "y2" <- w31
  "y1" <- w7
  n39 = Array Size(array=w25) -> (size(s)=w28:i32)
  "size(s)" <- w28
  n40 = call <vilib>:"Uniform White Noise.vi"("amplitude"="noise", "samples"=w28) -> ("uniform white noise"=w26:dbl[])  [unwired: 8 in, 1 out]
  n41 = Add(x=w25, y=w26) -> (x+y=w10:dbl[])
  "demodulated 2" <- w10
  "x+y" <- w10
  n42 = Array Size(array=w10) -> (size(s)=w14:i32)
  n43 = Divide(x=w28, y=w3) -> (x/y=w2:dbl)
  n44 = Increment(x=w2) -> (x+1=w1:dbl)
  n45 = for {
    N: w1 -> [_]
    tunnel: w7 -> [w118]
    tunnel: w31 -> [w107]
    tunnel: w10 -> [w105]
    shift-right: [w116] -> _
    shift-left: w3 -> [w106]
    tunnel: w3 -> [w117]
    tunnel: w3 -> [w100]
    tunnel: w30 -> [w90]
    tunnel: "bp (Bit Period)" -> [w103]
    tunnel: [w88] -> w15 mode=indexing
    w97 = 0.5 ("y")
    w104 = 2.0 ("y")
    n46 = Add(x=w117, y=w106) -> (x+y=w116:i32)
    n47 = Subtract(x=w106, y=w100) -> (x-y=w115:i32)
    n48 = Subtract(x=w106, y=w100) -> (x-y=w108:i32)
    n49 = Array Subset(array=w105, index=w115, length=w106) -> (w114:dbl[])
    n50 = Array Subset(array=w105, index=w108, length=w106) -> (w109:dbl[])
    n51 = Multiply(x=w118, y=w114) -> (x*y=w91:dbl[])
    n52 = Multiply(x=w107, y=w109) -> (x*y=w89:dbl[])
    n53 = call <vilib>:"Uneven Numeric Integration.vi"("T"=w90, "X"=w91) -> ("result"=w113:dbl)  [unwired: 8 in, 1 out]
    n54 = call <vilib>:"Uneven Numeric Integration.vi"("T"=w90, "X"=w89) -> ("result"=w110:dbl)  [unwired: 8 in, 1 out]
    n55 = Divide(x=w113, y=w103) -> (x/y=w112:dbl)
    n56 = Divide(x=w110, y=w103) -> (x/y=w111:dbl)
    n57 = Multiply(x=w112, y=w104) -> (x*y=w102:dbl)
    n58 = Multiply(x=w111, y=w104) -> (x*y=w101:dbl)
    n59 = Round To Nearest(number=w102) -> (nearest integer value=w99:dbl)
    n60 = Round To Nearest(number=w101) -> (nearest integer value=w98:dbl)
    n61 = Greater?(x=w98, y=w97) -> (0:w96:bool)
    n62 = Greater?(x=w99, y=w97) -> (0:w88:bool)
    n63 = Select(t=-1.0 ("y"), s=w96, f=0.0 ("y")) -> (s? t:f=w92:dbl)
    n64 = Select(t=1.0 ("y"), s=w88, f=w92) -> ()  [unwired: 1 out]
  }
  n65 = call <vilib>:"Sound Output Configure.vi"("number of samples/ch"=w14, "sample mode"=w23, "sound format"=T2 {"sample rate (S/s)"=44100.0, "number of channels"=1, "bits per sample"=16}, "device ID"=u32 0) -> ("task ID"=w22:T4)  [unwired: 6 in, 1 out]
  n66 = Tick Count (ms)() -> (millisecond timer value=w9:u32)
  n67 = while {
    tunnel: w22 -> [w122]
    tunnel: w10 -> [w124]
    tunnel: w9 -> [w120]
    stop <- FALSE stop-if-true
    n68 = call-poly <vilib>:"Sound Output Write.vi"("data"=w124, "task ID"=w122) -> ()  [unwired: 8 in, 2 out]
    n69 = Tick Count (ms)() -> (millisecond timer value=w121:u32)
    n70 = Subtract(x=w121, y=w120) -> (x-y=→"x-y":u32)
  }
  n71 = Initialize Array(TRUE, w3) -> (w19:bool[])
  n72 = Initialize Array(FALSE, w3) -> (w18:bool[])
  n73 = for {
    tunnel: w15 -> [w128] mode=indexing
    tunnel: w19 -> [w127]
    tunnel: w18 -> [w126]
    tunnel: [w125] -> w17 mode=concatenating
    n74 = Select(t=w127, s=w128, f=w126) -> (s? t:f=w125:bool[])
  }
  n75 = Boolean To (0,1)(Boolean=w17) -> (0, 1=w16:i16[])
  n76 = Build Array(w16, w11) -> (→"demodulated":i16[][])
